vi "AlliGator Save-Load IRFs & Fit Data (Map).vi"(8 "error in (no error)":errorcluster, 9 "Write(T)/Load (F)":bool, 10 "File Path":path, 11 "Data Value Reference in":refnum<data-value>) -> (0 "error out":errorcluster, 3 "Data Value Reference out":refnum<data-value>)   [LabVIEW 2021, in "AlliGator Decay Fit Parameter Map.lvlib"]
doc: "Load/Save Decay Fit Parameter Map & Metadata from/to HDF5 file."
uses:
  AlliGator Decay Fit Parameter Map.lvlib
  AlliGator Internal Variables v2.ctl
  <vilib>/vision/Image Controls.llb/IMAQ Image.ctl
  AlliGator Gate Image Set.ctl
  AlliGator FLI Dataset Type.ctl
  AlliGator Data Series Type.ctl
  AlliGator Dataset Channel.ctl
  AlliGator Gate Arithmetic.ctl
  AlliGator Displayed Image.ctl
  Image/Named ROI Description.ctl
  AlliGator Decay Metadata v3.ctl
  AlliGator Decay Background Subtraction Info.ctl
  AlliGator Baseline Subtraction Method.ctl
  Graphs/XY Graph/XY Graph Plot Shift Parameters.ctl
  Graphs/XY Graph/XY Graph Plot Shift Method.ctl
  AlliGator Decay Extrapolation Parameters.ctl
  Phasor/Calibration Phasor (m, phi).ctl
  Phasor/Phasor Reference Series.ctl
  Phasor/Phasor Calibration Map v2.ctl
  Phasor/Phasor (g, s).ctl
  AlliGator Raw Phasor Plot Data v4.ctl
  Phasor/Phasor Standard Deviation Options.ctl
  AlliGator Phasor Multi-Harmonic Data.ctl
  Phasor/Phasor Harmonic Data.ctl
  AlliGator Decay Fit Options & Parameters v2.ctl
  Fits/IRF(X)PSED/Decay Fit Options v2.ctl
  Fits/Decay Convolution/Decay Model.ctl
  Fits/Residual Type.ctl
  Fits/IRF(X)PSED/Fit Weights Type.ctl
  Fits/Non-linear Fitting Method v2.ctl
  Fits/Fit Calculation Method.ctl
  Fits/Non-linear Fitting Algorithm.ctl
  AlliGator Decay Fit Parameter Constraints 2.ctl
  Fits/IRF(X)PSED/Decay Fit Parameters In List.ctl
  Fits/IRF(X)PSED/MLE Baseline Offset Type.ctl
  AlliGator Decay Preprocessing Parameters.ctl
  Fits/IRF(X)PSED/Decay Fit Parameters & Derived Quantities List.ctl
  AlliGator IRFs & Fit Data v2.ctl
  AlliGator Globals.vi
  AlliGator Files.lvlib
  Fits/Fits.lvlib
  AlliGator Globals, Variables & Constants.lvlib
  Notebook/Notebook.lvlib
  Rich Text Box/Rich Text Box.lvlib
  Graphs/XY Graph/XY Graph Add-Ons.lvlib
  AlliGator Decay Preprocessing.lvlib
  Phasor/Phasor.lvlib
  Image/Image.lvlib
  AlliGator Phasor Graph.lvlib
  AlliGator Phasor Plot.lvlib
  AlliGator Source Image.lvlib
  AlliGator Internal Variables.lvlib
  AlliGator Decay Fit.lvlib
  AlliGator Settings.lvlib
  AlliGator Dual-Channel Datasets.lvlib
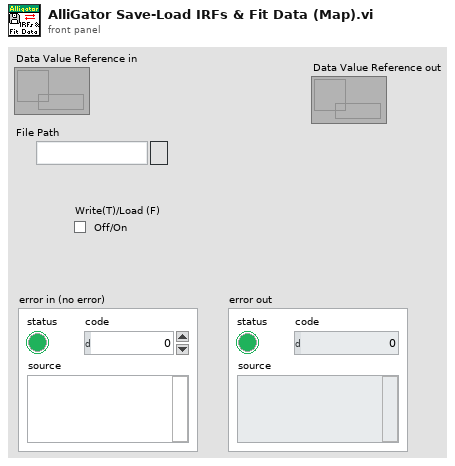
[diagram p1: front panel]
types:
  T1 = typedef "Fits.lvlib/Decay Model.ctl" = enum16{"1-Exponential", "2-Exponentials"}
  T2 = typedef "AlliGator Decay Fit Parameter Map.lvlib/AlliGator IRFs & Fit Data v2.ctl" = cluster{"IRF Array Time Axis":dbl[], "[IRFs]":dbl[][], "[Decay Fit Parameter Names]":T3[], "[Multiple Decays Fit Parameters]":dbl[][], "Fit Options: Decay Preprocessing Parameters":T4, "Fit Options: Reference Decay":cluster{"t Array":dbl[], "I Array":dbl[]}}
  T3 = typedef "Fits.lvlib/Decay Fit Parameters & Derived Quantities List.ctl" = enum16{"Offset", "Baseline", "A_1", "tau_1", "A_2", "tau_2", "<tau>_a", "f1_a", "f2_a", "<tau>_i", "f1_i", "f2_i", "-", "R^2", "Chi^2"}
  T4 = typedef "AlliGator Decay Analysis.lvlib/AlliGator Decay Preprocessing.lvlib/AlliGator Decay Preprocessing Parameters.ctl" = cluster{"Background Subtraction":bool, "Straighten Decay":bool, "Reverse Gates":bool, "1-Normalized Decay":bool, "Smoothen Decay":bool, "Smoothing Parameter":dbl, "Shift Decay":bool, "Decay Shift Parameters":T5, "Extrapolate Decay":bool, "Additional Points":u32, "Head Fraction":dbl, "Pixel-Normalize Decay":bool, "Use Periodicity":bool, "Use Cursors":bool, "Tail Fraction":dbl, "Use Decay Pre-Processing":bool, "Fold Decay":bool, "# Folds":u32, "[0-1]-Normalized Decay":bool}
  T5 = typedef "XY Graph Add-Ons.lvlib/XY Graph Plot Shift Parameters.ctl" = cluster{"Type":T6, "Shift":dbl[unit], "Threshold":dbl, "Rotate":bool}
  T6 = typedef "XY Graph Add-Ons.lvlib/XY Graph Plot Shift Method.ctl" = enum16{"Default", "CFD", "Threshold", "Cross-Correlation"}
  T7 = typedef "AlliGator Internal Variables.lvlib/AlliGator Internal Variables v2.ctl" = cluster{"Displayed Image":T8, "White Light Image":T8, "Mask Image":T8, "ROI Mask Image":T8, "Current Dataset Images 1":T9, "Background Dataset Images 1":T9, "Current Dataset Images 2":T9, "Background Dataset Images 2":T9, "Current Dataset Arithmetic Images":T9, "Accumulated Dataset Images 1":T9, "Accumulated Dataset Images 2":T9, "Accumulated Dataset Arithmetic Images":T9, "Phasor Plot Image":T8, "Decay Fit Parameter Map Image":T8, "Single Data Point Path":path, "White Light Image Path":path, "Mask Image Path":path, "Time-Series Folder":path, "[Time-Series Paths]":path[], "Current Dataset":i32, "Single Dataset Type":T10, "Current Folder":string, "AlliGator Data Series Type":T11, "# Datasets":i32, "Dual-Channel Dataset":bool, "Selected Channel Name":string, "Dataset Channel":T12, "Channel Arithmetic":T13, "Dual-Channel Background Dataset":bool, "Background Channel":T12, "Dual-Channel Accumulated Dataset":bool, "Start Time":dbl, "[Time-Series Timestamps]":dbl[], "[Intensity Corrections]":dbl[], "Time Series Script":bool, "Type of Displayed Image":T14, "Gate Image Slide":u16, "# Gates":i32, "ROIs":T15[], "ROI Decay":cluster{"t Array":dbl[], "I Array":dbl[]}, "Valid Decay":bool, "Decay  Metadata":T17, "Reference Decay Plot Name":string, "Reference Decay":cluster{"t Array":dbl[], "I Array":dbl[]}, "Decay Shift Plot":cluster{"Time Stamps":dbl[], "Decay Shifts":dbl[]}, "[Decays Max Values]":sgl[], "[Decays Min Values]":sgl[], "Calibration Phasor":T21, "Calibration Phasor Series":T22, "Phasor Calibration Map":T23, "Calibration Map MD5 Digest":string, "Last Raw Phasor":T24, "Last Calibrated Phasor":T24, "Last Calibrated Phasor SDV":T24, "Phasor Graph:Phasor Plot":cluster{"g Array":dbl[], "s Array":dbl[]}, "Phasor Graph:Phasor SDV Plot":cluster{"g Array":dbl[], "s Array":dbl[]}, "[Phasor Graph:Raw Phasor Plots]":T25[], "Phasor Plot locked to Ref 1":i32, "[Phasor Plot(s) locked to Ref 1]":i32[], "[Phasor Plot(s) locked to Ref 2]":i32[], "[Pixel Phasors]":T24[], "[[Sum Image]]":dbl[][], "[[CSG Phasors]]":csg[][], "[[Valid Pixel?]]":bool[][], "I/m/phi Dataset":cluster{"I/m/phi Dataset?":bool, "Base Frequency":dbl[unit], "Harmonic Orders":u8[]}, "Multi Phasor Plot Data":T27, "Decay Fit Options & Parameters":T29, "Fit Options: Decay Preprocessing Parameters":T4, "Fit Options: Reference Decay":cluster{"t Array":dbl[], "I Array":dbl[]}, "Is Full Image Parameters Map":bool, "Is Single-Pixels Parameters Map":bool, "NLSF Parameters Map X Resolution":i32, "NLSF Parameters Map Y Resolution":i32, "[Single Decay Fit Parameters]":dbl[], "Fit Model":T1, "[[Multiple Decays Fit Parameters]]":dbl[][], "[[Multiple Decays Fit Parameter SDVs]]":dbl[][], "[[IRFs]]":dbl[][], "IRF Array Time Axis":dbl[], "Decay Array Time Axis":dbl[], "[Decay Fit Parameter Names]":T3[], "[[Phasor Ratios]]":dbl[][], "[[Average Lifetimes]]":dbl[][], "Amplitude Weighted Average Lifetime":bool, "[Decay Sum]":dbl[], "[[User-defined Quantities]]":dbl[][], "User-defined Quantity":string}
  T8 = typedef "IMAQ Image.ctl" = refnum<image>
  T9 = typedef "AlliGator Internal Variables.lvlib/AlliGator Gate Image Set.ctl" = cluster{"SGL Image Max":T8, "SGL Image Sum":T8, "SGL Gate Images":T8[], "SGL Image Min":T8}
  T10 = typedef "AlliGator Files.lvlib/AlliGator FLI Dataset Type.ctl" = enum16{"HDF5 FLI Dataset", "Gate Image Folder", ".sdt FLI Dataset (Becker & Hickl)", ".ptu FLI Dataset (PicoQuant)", "SS1 FLI Dataset", "SS2 FLI Dataset", "I/m/phi Dataset", ".bin FLI Dataset (PicoQuant Binned)", ".bin FLI Dataset (Piccolo Binned)"}
  T11 = typedef "AlliGator Files.lvlib/AlliGator Data Series Type.ctl" = enum16{"Not a Supported Series", "Gate Images Folder Series", "SwissSPAD 2 Dataset Series", "B&H FLI Dataset Series", "PicoQuant PTU FLI Dataset Series", "PicoQuant BIN FLI Dataset Series", "Piccolo hist BIN FLI Dataset Series", "HDF5 FLI Dataset Series"}
  T12 = typedef "AlliGator Dual-Channel Datasets.lvlib/AlliGator Dataset Channel.ctl" = enum16{"G2", "INT"}
  T13 = typedef "AlliGator Settings.lvlib/AlliGator Gate Arithmetic.ctl" = enum16{"None", "INT-G2", "G2/INT*<INT>", "(1 - G2/INT)*<INT>"}
  T14 = typedef "AlliGator Source Image.lvlib/AlliGator Displayed Image.ctl" = enum16{"Single Gate", "Sum of All Gates", "Max of All Gates", "Min of All Gates", "-", "White Ligth Image", "Mask Image"}
  T15 = typedef "Image.lvlib/Named ROI Description.ctl" = cluster{"ROI Descriptor":T16, "ROI Name":string, "Overlay Color":u32}
  T16 = typedef "ROI Descriptor" = cluster{"Global Rectangle":i32[], "Contours":cluster{"ID":enum32{"External", "Internal"}, "Type":u32, "Coordinates":i32[]}[]}
  T17 = typedef "AlliGator Phasor Graph.lvlib/AlliGator Decay Metadata v3.ctl" = cluster{"ROI Descriptor":T16, "ROI Center":cluster{"X":i32, "Y":i32}, "Decay Background Subtraction Info":T18, "Decay Reverted":bool, "Decay Smoothened":bool, "Decay Straightened":bool, "Fitted Tau (Decay Straightening)":dbl, "Decay Shift Parameters":T5, "Decay Shifted":bool, "Decay Extrapolated":bool, "Decay Extrapolation Parameters":T20, "Decay Normalized":bool, "Fold Decay":bool, "# Folds":u32}
  T18 = typedef "AlliGator Decay Analysis.lvlib/AlliGator Decay Preprocessing.lvlib/AlliGator Decay Background Subtraction Info.ctl" = cluster{"Laser Period":dbl[unit], "Gate Duration":dbl[unit], "Baseline Subtraction Method":T19, "Background Definition Range":cluster{"Min Gate":dbl[unit], "Max Gate":dbl[unit]}, "Total Intensity w/o Bkgd Subtraction":dbl, "Bkgd-subtracted Intensity (exp)":dbl, "# Data Points":i32, "Background/Gate":dbl, "Fitted Lifetime":dbl[unit], "Bkgd-subtracted Intensity (theo)":dbl}
  T19 = typedef "AlliGator Decay Analysis.lvlib/AlliGator Decay Preprocessing.lvlib/AlliGator Baseline Subtraction Method.ctl" = enum16{"Mean", "Min", "Square Gated Single-Exponential", "File", "Constant"}
  T20 = typedef "AlliGator Decay Analysis.lvlib/AlliGator Decay Preprocessing.lvlib/AlliGator Decay Extrapolation Parameters.ctl" = cluster{"Additional Points":u32, "Head Fraction":dbl, "Fitted Tau":dbl, "Use Periodicity":bool, "Use Cursors":bool, "Tail Fraction":dbl}
  T21 = typedef "Phasor.lvlib/Calibration Phasor (m, phi).ctl" = cluster{"m":dbl, "phi":dbl, "Phasor Frequency":dbl[unit], "Reference Lifetime":dbl[unit]}
  T22 = typedef "Phasor.lvlib/Phasor Reference Series.ctl" = cluster{"m Array":dbl[], "phi Array":dbl[], "Phasor Frequency":dbl[unit], "Calibration Lifetime":dbl[unit]}
  T23 = typedef "Phasor.lvlib/Phasor Calibration Map v2.ctl" = cluster{"Phasor Frequency":dbl[unit], "Calibration Lifetime":dbl[unit], "ROI Centers":cluster{"X":i32, "Y":i32}[], "ROI Descriptors":T16[], "Map Resolution X":i32, "Map Resolution Y":i32, "z Array":cdb[]}
  T24 = typedef "Phasor.lvlib/Phasor (g, s).ctl" = cluster{"g":dbl, "s":dbl}
  T25 = typedef "AlliGator Phasor Graph.lvlib/AlliGator Raw Phasor Plot Data v4.ctl" = cluster{"Phasor Plot Name":string, "Raw Phasor Plot":T24[], "Phasor Frequency":dbl[unit], "[Decay Metadata]":T17[], "Raw Phasor Plot SDV":T24[], "Phasor SDV Options":T26, "[Calibration Phasor]":T21[]}
  T26 = typedef "Phasor.lvlib/Phasor Standard Deviation Options.ctl" = cluster{"Compute Estimated SDV":bool, "# Replicas":u32, "Use Estimated Average Phasor":bool}
  T27 = typedef "AlliGator Phasor Plot.lvlib/AlliGator Phasor Multi-Harmonic Data.ctl" = cluster{"Base Frequency":dbl[unit], "# Harmonics":u8, "Harmonic Orders":u8[], "Phasor Plot Settings Checksum":u64, "Phasor Harmonic Data Array":T28[]}
  T28 = typedef "Phasor.lvlib/Phasor Harmonic Data.ctl" = cluster{"Phasor Harmonic Name":string, "Phasor Plot Settings Checksum":u64, "Phasor Frequency":dbl[unit], "Base Frequency":dbl[unit], "Harmonic Order":u8, "Phasor Plot Parameters":string, "Phasor Array [[CSG]]":csg[][], "Dataset File Path":path}
  T29 = typedef "AlliGator Decay Fit Parameter Map.lvlib/AlliGator Decay Fit Options & Parameters v2.ctl" = cluster{"SYNC Period":dbl[unit], "Fit Options":T30, "Fit Parameter Constraints":T36[], "MLE Baseline Offset":dbl, "MLE Baseline Offset Type":T38}
  T30 = typedef "Fits.lvlib/Decay Fit Options v2.ctl" = cluster{"Show Fit Residuals":bool, "Fit Model":T1, "Residual Type":T31, "Max Decay Percentile":dbl, "Min Decay Percentile":dbl, "Show Full Decay":bool, "Weights":T32, "Fitting Method":T33, "Compute Parameter Uncertainties":bool, "Periodic Boundaries":bool, "Model Calculation":T34, "Period":dbl[unit], "Termination Criteria":cluster{"Max Iterations":i32, "Max Function Calls":i32, "Max Time":dbl[unit], "Function Tolerance":dbl, "Parameter Tolerance":dbl, "Gradient Tolerance":dbl, "Min Lambda":dbl, "Max Lambda":dbl, "Initial Tick Count":u32}, "Offset Resolution":dbl[unit], "Use Local IRF":bool, "Fitting Algorithm":T35}
  T31 = typedef "Fits.lvlib/Residual Type.ctl" = enum16{"Standard", "Normalized", "Reduced"}
  T32 = typedef "Fits.lvlib/Fit Weights Type.ctl" = enum16{"Unweighted", "1/Variance", "Best of All"}
  T33 = typedef "Fits.lvlib/Non-linear Fitting Method v2.ctl" = enum16{"Least Square", "Least Absolute Residual", "Bisquare", "MLE", "-", "Best of All"}
  T34 = typedef "Fits.lvlib/Fit Calculation Method.ctl" = enum16{"Simulation", "Convolution", "Integration"}
  T35 = typedef "Fits.lvlib/Non-linear Fitting Algorithm.ctl" = enum16{"Levenberg-Marquardt", "Trust-Region Dogleg"}
  T36 = typedef "AlliGator Decay Analysis.lvlib/AlliGator Decay Fit.lvlib/AlliGator Decay Fit Parameter Constraints 2.ctl" = cluster{"Fit Parameter":T37, "Min Value":dbl, "Max Value":dbl, "Global":bool, "Used":bool}
  T37 = typedef "Fits.lvlib/Decay Fit Parameters In List.ctl" = enum16{"Offset", "Baseline", "A_1", "tau_1", "A_2", "tau_2"}
  T38 = typedef "Fits.lvlib/MLE Baseline Offset Type.ctl" = enum32{"Absolute", "Percentage"}
  T39 = typedef "AlliGator Decay Fit Parameter Map.lvlib/AlliGator IRFs & Fit Data v1.ctl" = cluster{"IRF Array Time Axis":dbl[], "[IRF]":dbl[][], "[Decay Fit Parameter Name]":T3[], "[Multiple Decays Fit Parameters]":dbl[][]}
  T40 = typedef "Rich Text Box.lvlib/Text Formatting.ctl" = cluster{"Font":string, "Text Color":T41, "Text Background Color":T41, "Text Style":enum16{"Regular", "Bold", "Italic", "Underline", "Strikeout"}, "Font Size (Points)":dbl, "Text Alignment":i32}
  T41 = typedef "Rich Text Box.lvlib/Text Colors.ctl" = enum16{"Unchanged", "Black", "Blue", "Brown", "Gray", "Green", "Orange", "Pink", "Red", "White"}
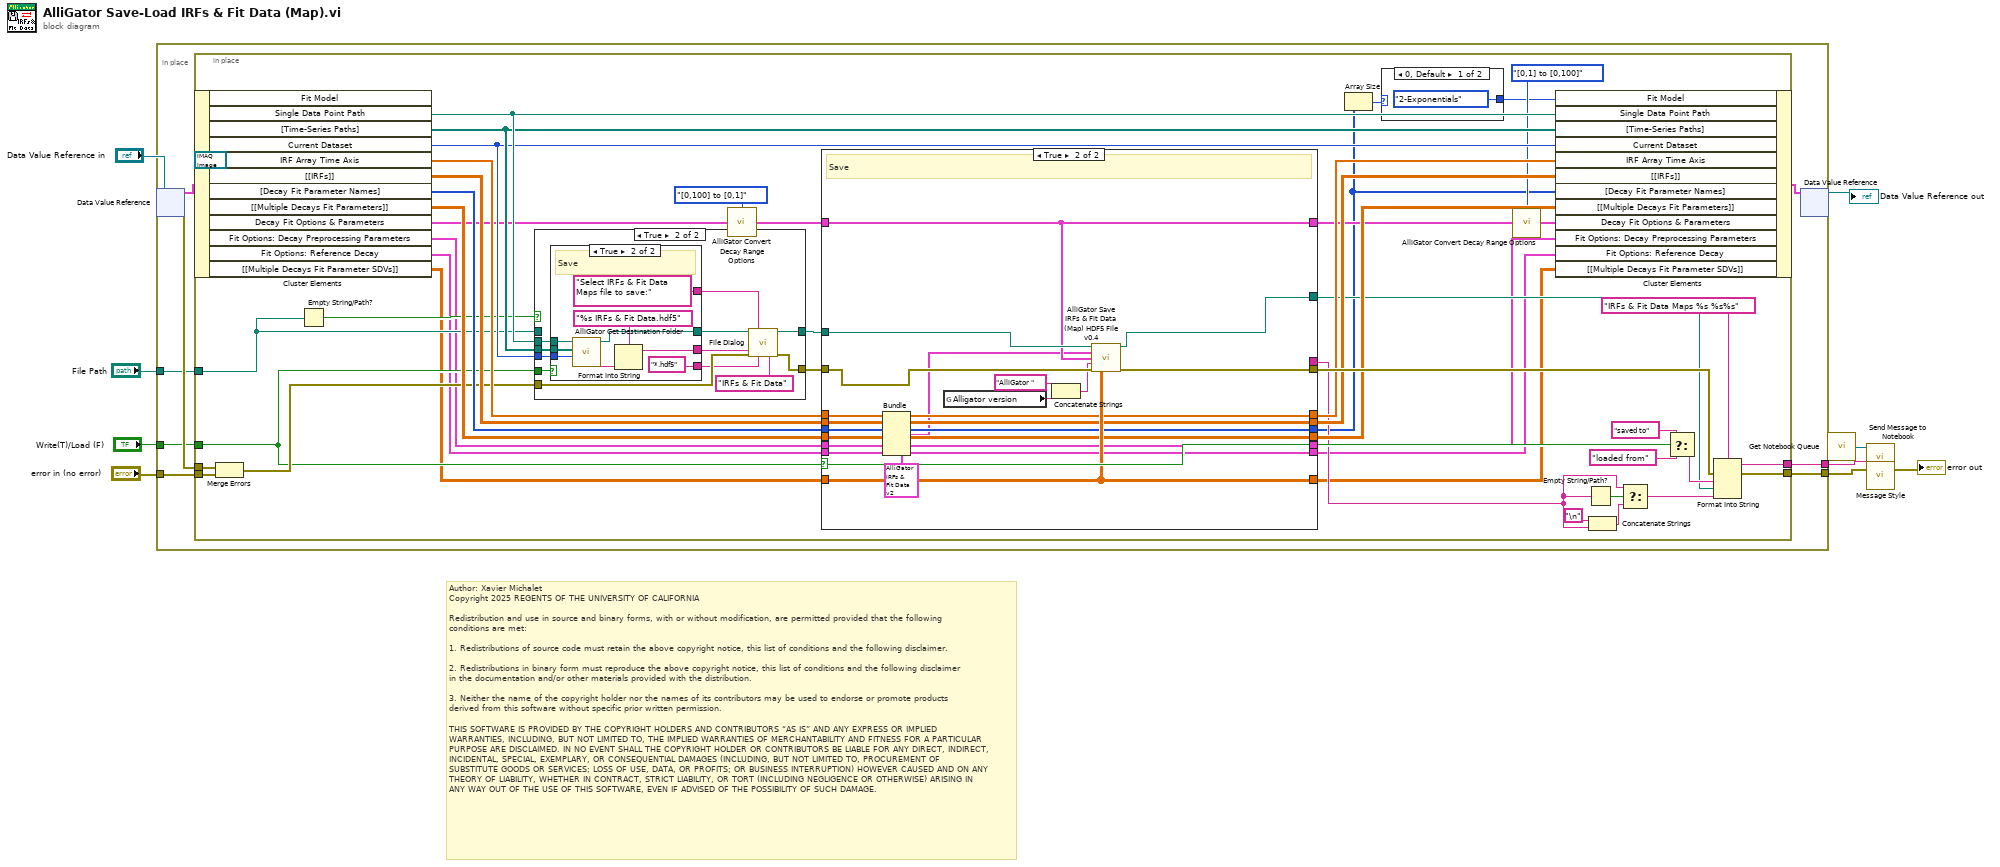
[diagram p0: block diagram]
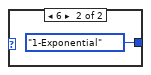
[diagram p2: hidden frame]
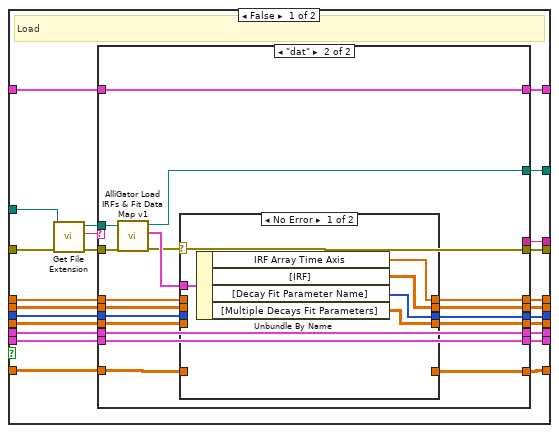
[diagram p3: hidden frame]
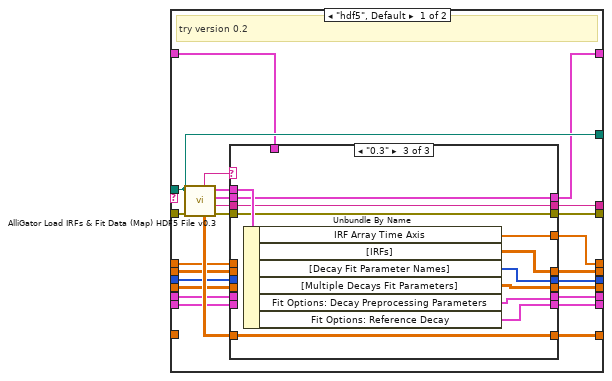
[diagram p4: hidden frame]
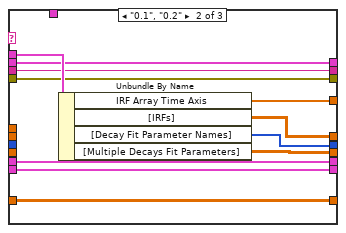
[diagram p6: hidden frame]
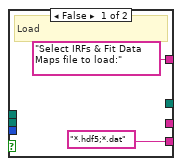
[diagram p9: hidden frame]
diagram:
  # "Author: Xavier Michalet\nCopyright 2025 REGENTS OF THE UNIVERSITY OF CALIFORNIA\n\nRedistribution and use in source and binary forms, with or without modification, are permitted provided that the following conditions are met:\n\n1. Redistributions of source code must retain the above copyright notice, this list of conditions and the following disclaimer.\n\n2. Redistributions in binary form must reproduce the above copyright notice, this list of conditions and the following disclaimer in the documentation and/or other materials provided with the distribution.\n\n3. Neither the name of the copyright holder nor the names of its contributors may be used to endorse or promote products derived from this software without specific prior written permission.\n\nTHIS SOFTWARE IS PROVIDED BY THE COPYRIGHT HOLDERS AND CONTRIBUTORS “AS IS” AND ANY EXPRESS OR IMPLIED WARRANTIES, INCLUDING, BUT NOT LIMITED TO, THE IMPLIED WARRANTIES OF MERCHANTABILITY AND FITNESS FOR A PARTICULAR PURPOSE ARE DISCLAIMED. IN NO EVENT SHALL THE COPYRIGHT HOLDER OR CONTRIBUTORS BE LIABLE FOR ANY DIRECT, INDIRECT, INCIDENTAL, SPECIAL, EXEMPLARY, OR CONSEQUENTIAL DAMAGES (INCLUDING, BUT NOT LIMITED TO, PROCUREMENT OF SUBSTITUTE GOODS OR SERVICES; LOSS OF USE, DATA, OR PROFITS; OR BUSINESS INTERRUPTION) HOWEVER CAUSED AND ON ANY THEORY OF LIABILITY, WHETHER IN CONTRACT, STRICT LIABILITY, OR TORT (INCLUDING NEGLIGENCE OR OTHERWISE) ARISING IN ANY WAY OUT OF THE USE OF THIS SOFTWARE, EVEN IF ADVISED OF THE POSSIBILITY OF SUCH DAMAGE."
  n1 = in-place {
    in-place-border: "error in (no error)" -> [w16]
    in-place-border: [w14] -> w2
    in-place-border: [w13] -> w3
    in-place-border: "Write(T)/Load (F)" -> [w12]
    in-place-border: "File Path" -> [w11]
    n2 = in-place-dvr #1("Data Value Reference in") -> (w18:T7, w15:errorcluster)
    n3 = in-place {
      in-place-border: w16 -> [w64]
      in-place-border: w15 -> [w60]
      in-place-border: [w58] -> w14
      in-place-border: [w57] -> w13
      in-place-border: w12 -> [w38]
      in-place-border: w11 -> [w43]
      (unwired) T8 refnum ("Current Dataset Images.Image Sum")
      n4 = in-place-cluster #2(w18) -> ("Single Data Point Path"=w63:path, "[Time-Series Paths]"=w62:path[], "Current Dataset"=w61:i32, "IRF Array Time Axis"=w52:dbl[], "[[IRFs]]"=w51:dbl[][], "[Decay Fit Parameter Names]"=w50:T3[], "[[Multiple Decays Fit Parameters]]"=w49:dbl[][], "Decay Fit Options & Parameters"=w39:T29, "Fit Options: Decay Preprocessing Parameters"=w30:T4, "Fit Options: Reference Decay"=w29:cluster{"t Array":dbl[], "I Array":dbl[]}, "[[Multiple Decays Fit Parameter SDVs]]"=w32:dbl[][])  [unwired: 1 out]
      n5 = Merge Errors(w60, w64) -> (w42:errorcluster)
      n6 = Empty String/Path?(string/path=w43) -> (empty?=w44:bool)
      n7 = case shown="True" w44 {
        tunnel: w63 -> [_ w205]
        tunnel: w62 -> [_ w204]
        tunnel: w61 -> [_ w203]
        tunnel: w43 -> [w193 _]
        tunnel: w42 -> [w192 w200]
        tunnel: [w193 w199] -> w41
        tunnel: [w192 w198] -> w40
        tunnel: w38 -> [_ w196]
        frame False {
        }
        frame True {
          n8 = case shown="True" w196 {
            tunnel: w205 -> [_ w216]
            tunnel: w204 -> [_ w215]
            tunnel: w203 -> [_ w214]
            tunnel: [_ w211] -> w202
            tunnel: [_ w210] -> w201
            tunnel: ["Select IRFs & Fit Data Maps file to load:" ("prompt") "Select IRFs & Fit Data Maps file to save:" ("prompt")] -> w195
            tunnel: ["*.hdf5;*.dat" ("pattern (all files)") "*.hdf5" ("pattern (all files)")] -> w194
            frame False {
              # "Load"
            }
            frame True {
              # "Save"
              n9 = call "AlliGator Get Destination Folder.vi"("Current Data Set (-1: single)"=w214, "Time-Series Paths"=w215, "Single Data Point Path"=w216) -> ("Data Point Name"=w213:string, "Destination Folder path"=w211:path)  [unwired: 6 in, 1 out]
              n10 = Format Into String(format string="%s IRFs & Fit Data.hdf5", w213) -> (resulting string=w210:string)  [unwired: 2 in, 1 out]
            }
          }
          n11 = call "File Dialog"("start path"=w202, "prompt"=w195, "default name"=w201, "error in"=w200, "pattern (all files)"=w194, "pattern label"="IRFs & Fit Data") -> ("selected path"=w199:path, "error out"=w198:errorcluster)  [unwired: 6 in, 2 out]
        }
      }
      n12 = call "AlliGator Convert Decay Range Options.vi"("Decay Fit Options & Parameters in"=w39, "Percentile Conversion"=enum32{"[0,1] to [0,100]", "[0,100] to [0,1]"}."[0,100] to [0,1]") -> ("Decay Fit Options & Parameters out"=w26:T29)
      n13 = case shown="True" w38 {
        tunnel: [w82 w190] -> w59
        tunnel: [w81 w191] -> w45
        tunnel: w52 -> [w86 w185]
        tunnel: w51 -> [w85 w184]
        tunnel: w50 -> [w84 w183]
        tunnel: w49 -> [w83 w182]
        tunnel: [w90 w185] -> w48
        tunnel: [w89 w184] -> w47
        tunnel: [w88 w183] -> w21
        tunnel: [w87 w182] -> w46
        tunnel: w41 -> [w80 w189]
        tunnel: w40 -> [w78 w188]
        tunnel: w26 -> [w74 w187]
        tunnel: [w75 w187] -> w24
        tunnel: [w73 _] -> w35
        tunnel: w32 -> [w71 w186]
        tunnel: [w72 w186] -> w31
        tunnel: w30 -> [w70 w181]
        tunnel: w29 -> [w68 w180]
        tunnel: [w69 w181] -> w28
        tunnel: [w67 w180] -> w27
        frame False {
          # "Load"
          n14 = call <vilib>:"Get File Extension.vi"("error in (no error)"=w78, "file"=w80) -> ("error out"=w79:errorcluster, "lowercase file extension"=w77:string, "dup file"=w76:path)  [unwired: 5 in, 2 out]
          n15 = case shown="\"dat\"" w77 {
            tunnel: [w113 w163] -> w90
            tunnel: [w112 w162] -> w89
            tunnel: [w111 w161] -> w88
            tunnel: [w110 w160] -> w87
            tunnel: w86 -> [w95 w159]
            tunnel: w85 -> [w94 w158]
            tunnel: w84 -> [w93 w157]
            tunnel: w83 -> [w92 w156]
            tunnel: [w108 w155] -> w82
            tunnel: [w107 w154] -> w81
            tunnel: w79 -> [w115 w153]
            tunnel: w76 -> [w107 w152]
            tunnel: [w102 w151] -> w75
            tunnel: w74 -> [w91 w151]
            tunnel: [w101 _] -> w73
            tunnel: [w103 w149] -> w72
            tunnel: w71 -> [_ w150]
            tunnel: w70 -> [w99 w148]
            tunnel: [w98 w148] -> w69
            tunnel: w68 -> [w97 w147]
            tunnel: [w96 w147] -> w67
            frame "hdf5", Default {
              # "try version 0.2"
              n16 = call "AlliGator Load IRFs & Fit Data (Map) HDF5 File v0.3.vi"("Error In"=w115, "File Path"=w107) -> ("error out"=w109:errorcluster, "Data Description"=w105:string, "Decay Fit Options & Parameters"=w106:T29, "IRFs & Fit Data Map"=w114:T2, "[Multiple Decays Fit Parameters SDV]"=w104:dbl[][], "File Version"=w100:string)  [unwired: 3 in, 1 out]
              n17 = case shown="\"0.3\"" w100 {
                tunnel: w114 -> [_ w135 w146]
                tunnel: [w124 w134 w145] -> w113
                tunnel: [w123 w133 w144] -> w112
                tunnel: [w122 w132 w143] -> w111
                tunnel: [w121 w131 w142] -> w110
                tunnel: [w117 w130 w141] -> w108
                tunnel: w106 -> [_ w128 w139]
                tunnel: w105 -> [_ w127 w138]
                tunnel: w104 -> [w118 w129 w140]
                tunnel: [w118 w129 w140] -> w103
                tunnel: [w116 w128 w139] -> w102
                tunnel: [_ w127 w138] -> w101
                tunnel: w109 -> [w117 w130 w141]
                tunnel: [w120 w126 w137] -> w98
                tunnel: w99 -> [w120 w126 _]
                tunnel: w97 -> [w119 w125 _]
                tunnel: [w119 w125 w136] -> w96
                tunnel: w95 -> [w124 _ _]
                tunnel: w94 -> [w123 _ _]
                tunnel: w93 -> [w122 _ _]
                tunnel: w92 -> [w121 _ _]
                tunnel: w91 -> [w116 _ _]
                frame Default {
                }
                frame "0.1", "0.2" {
                  n18 = Unbundle By Name(w135) -> ("IRF Array Time Axis"=w134:dbl[], "[IRFs]"=w133:dbl[][], "[Decay Fit Parameter Names]"=w132:T3[], "[Multiple Decays Fit Parameters]"=w131:dbl[][])
                }
                frame "0.3" {
                  n19 = Unbundle By Name(w146) -> ("IRF Array Time Axis"=w145:dbl[], "[IRFs]"=w144:dbl[][], "[Decay Fit Parameter Names]"=w143:T3[], "[Multiple Decays Fit Parameters]"=w142:dbl[][], "Fit Options: Decay Preprocessing Parameters"=w137:T4, "Fit Options: Reference Decay"=w136:cluster{"t Array":dbl[], "I Array":dbl[]})
                }
              }
            }
            frame "dat" {
              n20 = call "AlliGator Load IRFs & Fit Data Map v1.vi"("error in (no error)"=w153, "File Path in"=w152) -> ("error out"=w155:errorcluster, "IRFs & Fit  Data Map"=w164:T39, "File Path out"=w154:path)  [unwired: 7 in]
              n21 = case shown="No Error" w155 {
                tunnel: w164 -> [w169 _]
                tunnel: [w168 w174] -> w163
                tunnel: [w167 w173] -> w162
                tunnel: [w166 w172] -> w161
                tunnel: [w165 w171] -> w160
                tunnel: w159 -> [_ w174]
                tunnel: w158 -> [_ w173]
                tunnel: w157 -> [_ w172]
                tunnel: w156 -> [_ w171]
                tunnel: w150 -> [_ w170]
                tunnel: [_ w170] -> w149
                frame No Error {
                  n22 = Unbundle By Name(w169) -> ("IRF Array Time Axis"=w168:dbl[], "[IRF]"=w167:dbl[][], "[Decay Fit Parameter Name]"=w166:T3[], "[Multiple Decays Fit Parameters]"=w165:dbl[][])
                }
                frame Error {
                }
              }
            }
          }
        }
        frame True {
          # "Save"
          n23 = Bundle(cluster=T2 {"IRF Array Time Axis"=[], "[IRFs]"=[], "[Decay Fit Parameter Names]"=[], "[Multiple Decays Fit Parameters]"=[], "Fit Options: Decay Preprocessing Parameters"={"Background Subtraction"=FALSE, "Straighten Decay"=FALSE, "Reverse Gates"=FALSE, "1-Normalized Decay"=FALSE, "Smoothen Decay"=FALSE, "Smoothing Parameter"=0.0, "Shift Decay"=FALSE, "Decay Shift Parameters"={"Type"=enum."Default", "Shift"=0.0, "Threshold"=0.0, "Rotate"=FALSE}, "Extrapolate Decay"=FALSE, "Additional Points"=0, "Head Fraction"=0.0, "Pixel-Normalize Decay"=FALSE, "Use Periodicity"=FALSE, "Use Cursors"=FALSE, "Tail Fraction"=0.0, "Use Decay Pre-Processing"=FALSE, "Fold Decay"=FALSE, "# Folds"=0, "[0-1]-Normalized Decay"=FALSE}, "Fit Options: Reference Decay"={"t Array"=[], "I Array"=[]}} ("output cluster"), "IRF Array Time Axis"=w185, "[IRFs]"=w184, "[Decay Fit Parameter Names]"=w183, "[Multiple Decays Fit Parameters]"=w182, "Fit Options: Decay Preprocessing Parameters"=w181, "Fit Options: Reference Decay"=w180) -> (w175:T2)
          n24 = global read "AlliGator Globals.vi" "Alligator version"() -> (w179:string)
          n25 = Concatenate Strings("AlliGator " ("string"), w179) -> (w177:string)
          n26 = call "AlliGator Save IRFs & Fit Data (Map) HDF5 File v0.4.vi"("File Path"=w189, "IRFs & Fit Data Map v2"=w175, "Decay Fit Options & Parameters"=w187, "Software + Version"=w177, "Error In"=w188, "[Multiple Decays Fit Parameters SDV]"=w186) -> ("File Path out"=w191:path, "Error Out"=w190:errorcluster)  [unwired: 7 in, 1 out]
        }
      }
      n27 = Array Size(array=w21) -> (size(s)=w20:i32)
      n28 = case shown="0, Default" w20 {
        tunnel: [Decay_Model."2-Exponentials" ("Fit Model") Decay_Model."1-Exponential" ("Fit Model")] -> w19
        frame 0, Default {
        }
        frame 6 {
        }
      }
      n29 = call "AlliGator Convert Decay Range Options.vi"("Decay Fit Options & Parameters in"=w24, "Percentile Conversion"=enum32{"[0,1] to [0,100]", "[0,100] to [0,1]"}."[0,1] to [0,100]") -> ("Decay Fit Options & Parameters out"=w23:T29)
      n30 = in-place-cluster #2("Fit Model"=w19, "Single Data Point Path"=w63, "[Time-Series Paths]"=w62, "Current Dataset"=w61, "IRF Array Time Axis"=w48, "[[IRFs]]"=w47, "[Decay Fit Parameter Names]"=w21, "[[Multiple Decays Fit Parameters]]"=w46, "Decay Fit Options & Parameters"=w23, "Fit Options: Decay Preprocessing Parameters"=w28, "Fit Options: Reference Decay"=w27, "[[Multiple Decays Fit Parameter SDVs]]"=w31) -> (w17:T7)
      n31 = Empty String/Path?(string/path=w35) -> (empty?=w37:bool)
      n32 = Concatenate Strings("\n", w35) -> (w33:string)
      n33 = Select(t=w35, s=w37, f=w33) -> (s? t:f=w36:string)
      n34 = Select(t="saved to" ("format string"), s=w38, f="loaded from" ("format string")) -> (s? t:f=w53:string)
      n35 = Format Into String(format string="IRFs & Fit Data Maps %s %s%s", error in=w59, w53, w45, w36) -> (resulting string=w57:string, error out=w58:errorcluster)  [unwired: 1 in]
    }
    n36 = in-place-dvr #1(w17) -> (→"Data Value Reference out":refnum<data-value>)  [unwired: 1 out]
  }
  n37 = call "Get Notebook Queue.vi"() -> ("Notebook Queue"=w4:refnum<queue>)  [unwired: 9 in]
  n38 = call "Message Style.vi"() -> ("Message Formatting"=w5:T40)
  n39 = call "Send Message to Notebook.vi"("Text Formatting"=w5, "Error In"=w2, "Message"=w3, "Notebook Queue"=w4) -> ("Error Out"=→"error out":errorcluster)  [unwired: 4 in, 1 out]
